vi "Update_Analized_CoorOverlay.vi"(4 "Index":i32, 5 "DLL/Vision":bool, 6 "Listbox In":string[][](array[string]), 7 "ROI Entry":T10={"vROIName"="", "vROIContour"={"Contour Type"=0, "ROI Type"=0, "Points"=[]}, "ProcessSetting"=[], "Analysis_Setting"={"PreProcess"=enum."*Algorithm*", "Parameter"=""}}, 8 "error in (no error)":errorcluster, 9 "Available Points In":refnum<vi>, 10 "AnalysisResult":variant, 11 "Image Refnum":refnum<vi>) -> (0 "error out":errorcluster, 3 "Listbox Out":string[][](array[string]))   [LabVIEW 2019]
uses:
  Control/CoordinateAnalysisSetting.ctl
  DLL/[Global] Image.vi
  Analysis/Controls/Parttern Match/Analysis_PatternMatch_ResultWithnumber.ctl
  Process/Controls/Process_Setting.ctl
  Analysis/Controls/Analysis_Setting.ctl
  Controls/Vision_DataEntry.ctl
  <vilib>/vision/Measure.llb/Edge New.ctl
  <vilib>/vision/Image Controls.llb/IMAQ Image.ctl
  Ctrl/VisionProcessName.ctl
panel:
  out "DLL Vision_Image":T1
  in  "Particle output cluster":T2
  in  "Clamp MAX output cluster":T3
  in  "Clamp output cluster":T5 {"?"."Rectangle"."Rotation" format="%.2f"; "?"."Rectangle"."Left" scale=0.0..1024.0; "?"."Rectangle"."Right" scale=0.0..1024.0}
  in  "Barcode 1D output cluster":T6
  in  "Edge Detectionoutput cluster":T8 {"?"."Edge Information"."Distance (Real-World)" format="%.2f"; "?"."Edge Information"."Location (Real-World)"."Y" format="%.2g"; "?"."Edge Information"."Location (Real-World)"."X" format="%.2f"; "?"."Edge Information"."Noise" format="%.2f"; "?"."Edge Information"."Location (Pixel)"."Y" format="%.2g"; "?"."Edge Information"."Location (Pixel)"."X" format="%.2f"; "?"."Edge Information"."Strength" format="%.2f"; "?"."Edge Information"."Distance (Pixel)" format="%.2f"}
  in  "Barcode 2D output cluster":T9
  in  "Vision_Image":T1(plugin-control)
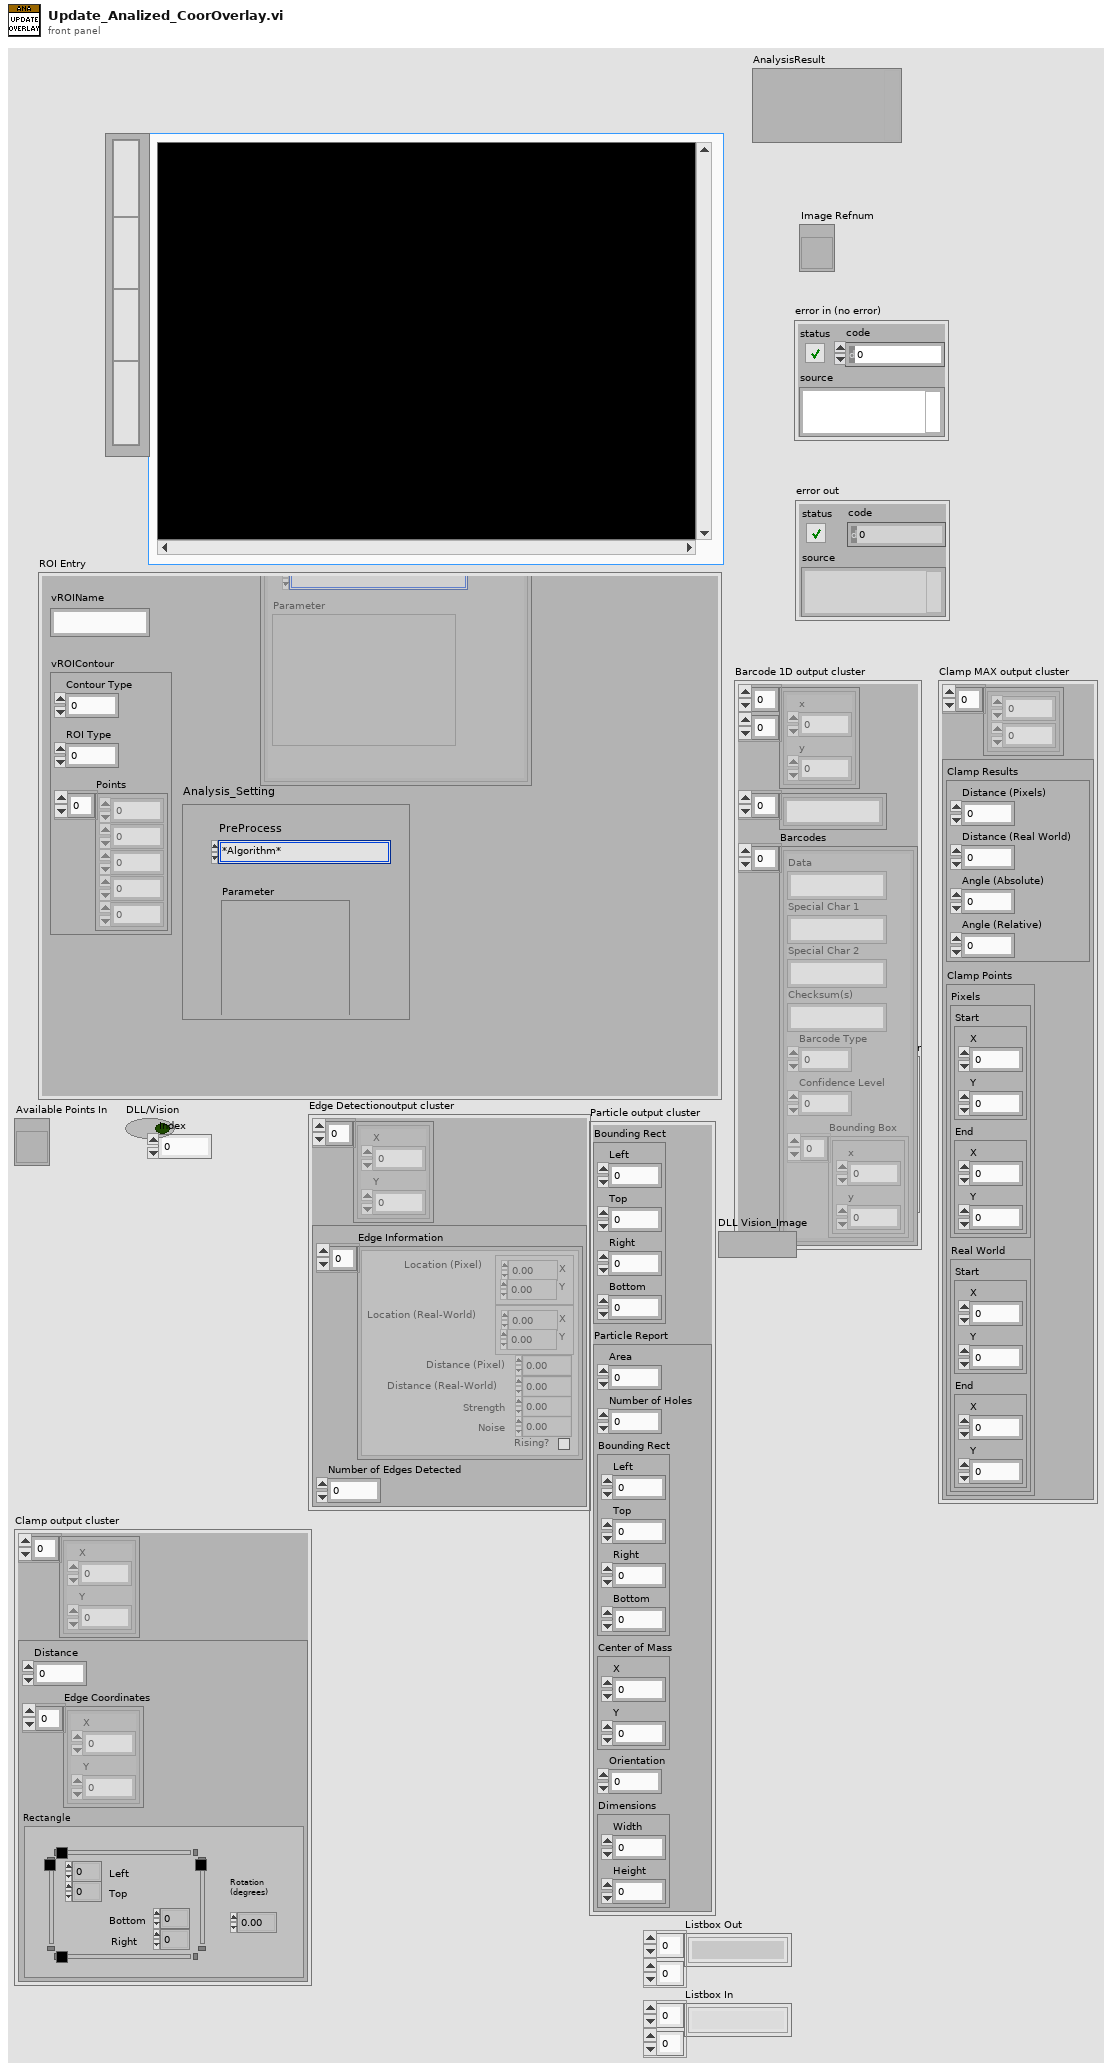
[diagram p1: front panel]
types:
  T1 = typedef "IMAQ Image.ctl" = refnum<image>
  T2 = cluster{"Bounding Rect":cluster{"Left":dbl, "Top":dbl, "Right":dbl, "Bottom":dbl}, "Particle Report":cluster{"Area":dbl, "Number of Holes":dbl, "Bounding Rect":cluster{"Left":dbl, "Top":dbl, "Right":dbl, "Bottom":dbl}, "Center of Mass":cluster{"X":dbl, "Y":dbl}, "Orientation":dbl, "Dimensions":cluster{"Width":dbl, "Height":dbl}}}
  T3 = cluster{cluster{dbl, dbl}[], cluster{"Clamp Results":cluster{"Distance (Pixels)":dbl, "Distance (Real World)":dbl, "Angle (Absolute)":dbl, "Angle (Relative)":dbl}, "Clamp Points":cluster{"Pixels ":cluster{"Start":cluster{"X":dbl, "Y":dbl}, "End":cluster{"X":dbl, "Y":dbl}}, "Real World":cluster{"Start":cluster{"X":dbl, "Y":dbl}, "End":cluster{"X":dbl, "Y":dbl}}}}}
  T4 = typedef "IMAQ Rectangle" = cluster{"Left":i32, "Top":i32, "Right":i32, "Bottom":i32, "Rotation":dbl}
  T5 = cluster{cluster{"X":sgl, "Y":sgl}[], cluster{"Distance":sgl, "Edge Coordinates":cluster{"X":sgl, "Y":sgl}[], "Rectangle":T4}}
  T6 = cluster{cluster{"x":sgl, "y":sgl}[][], string[], "Barcodes":cluster{"Data":string, "Special Char 1":string, "Special Char 2":string, "Checksum(s)":string, "Barcode Type":u32, "Confidence Level":sgl, "Bounding Box":cluster{"x":sgl, "y":sgl}[]}[]}
  T7 = typedef "Edge New.ctl" = cluster{"Location (Pixel)":cluster{"X":sgl, "Y":sgl}, "Location (Real-World)":cluster{"X":sgl, "Y":sgl}, "Distance (Pixel)":dbl, "Distance (Real-World)":dbl, "Strength":dbl, "Noise":dbl, "Rising?":bool}
  T8 = cluster{cluster{"X":sgl, "Y":sgl}[], cluster{"Edge Information":T7[], "Number of Edges Detected":i32}}
  T9 = cluster{"Data":string, cluster{"x":sgl, "y":sgl}[]}
  T10 = typedef "Vision_DataEntry.ctl" = cluster{"vROIName":string, "vROIContour":cluster{"Contour Type":u32, "ROI Type":u32, "Points":i32[]}, "ProcessSetting":T11[], "Analysis_Setting":T13}
  T11 = typedef "Process_Setting.ctl" = cluster{"Enum_PreProcess":T12, "Parameter":string}
  T12 = typedef "VisionProcessName.ctl" = enum16{"*CamParameter*", "CamAttributes", "*Preprocess*", "CG_Brightness", "C_Plane Extraction", "C_Threshold", "G_Lookup Table", "G_Threshold"}
  T13 = typedef "Analysis_Setting.ctl" = cluster{"PreProcess":T14, "Parameter":string}
  T14 = typedef "VisionProcessName.ctl" = enum16{"*CamParameter*", "CamAttributes", "*Preprocess*", "CG_Brightness", "C_Plane Extraction", "C_Threshold", "G_Lookup Table", "G_Threshold", "B_Image Inversion", "*Algorithm*", "CG_Histogram", "C_Color Matching", "C_Color Pattern Matching", "G_PatternMatch", "CG_Find Straight Edge", "CG_Adv. Find Straight Edge", "CG_Find Circular Edge", "G_Max Clamp", "G_Clamp (Rake)", "G_Pattern Matching"}
  T15 = typedef "CoordinateAnalysisSetting.ctl" = cluster{"Analysis_Type":enum16{"PatternMatch", "Straight Edge"}, "ROI ":T16, "Parameter":variant, "Step Result":variant, "AnalysisStepName":string, "CoordinateUse":bool}
  T16 = typedef "ROI Descriptor" = cluster{"Global Rectangle":i32[], "Contours":cluster{"ID":enum32{"External", "Internal"}, "Type":u32, "Coordinates":i32[]}[]}
  T17 = typedef "Analysis_Type.ctl" = u16
  T18 = typedef "Analysis_PatternMatch_ResultWithnumber.ctl" = cluster{"numbers":i32, "results":cluster{"ROI Descriptor out":T16, "Point":T19, "Angle":sgl, "Score":sgl, "Real World Coordinates":cluster{"X":sgl, "Y":sgl}, "Rectangle":T4}[]}
  T19 = typedef "IMAQ Point" = cluster{"X":sgl, "Y":sgl}
  T20 = cluster{"Point1 (Pixels)":cluster{"X":sgl, "Y":sgl}, "Point2 (Pixels)":cluster{"X":sgl, "Y":sgl}, "Point1 (Real-World)":cluster{"X":sgl, "Y":sgl}, "Point2 (Real-World)":cluster{"X":sgl, "Y":sgl}, "Angle (Pixel)":dbl, "Angle (Real-World)":dbl, "Score":dbl, "Straightness":dbl, "Average SNR (db)":dbl, "Calibration Valid":bool}[]
  T21 = cluster{"ROI Descriptor out":T16, "Point":T19, "Angle":sgl, "Score":sgl, "Real World Coordinates":cluster{"X":sgl, "Y":sgl}, "Rectangle":T4}[]
  T22 = cluster{"Left":dbl, "Top":dbl, "Right":dbl, "Bottom":dbl}
  T23 = cluster{"ROI Descriptor out":cluster{"Global Rectangle":i32[], "Contours":cluster{"ID":enum32{"External", "Internal"}, "Type":u32, "Coordinates":i32[]}[]}, "Output value":dbl}
  T24 = cluster{"Global Rectangle":i32[], "Contours":cluster{"ID":enum32{"External", "Internal"}, "Type":u32, "Coordinates":i32[]}[]}
  T25 = cluster{"ID":enum32{"External", "Internal"}, "Type":u32, "Coordinates":i32[]}[]
  T26 = cluster{"ID":enum32{"External", "Internal"}, "Type":u32, "Coordinates":i32[]}
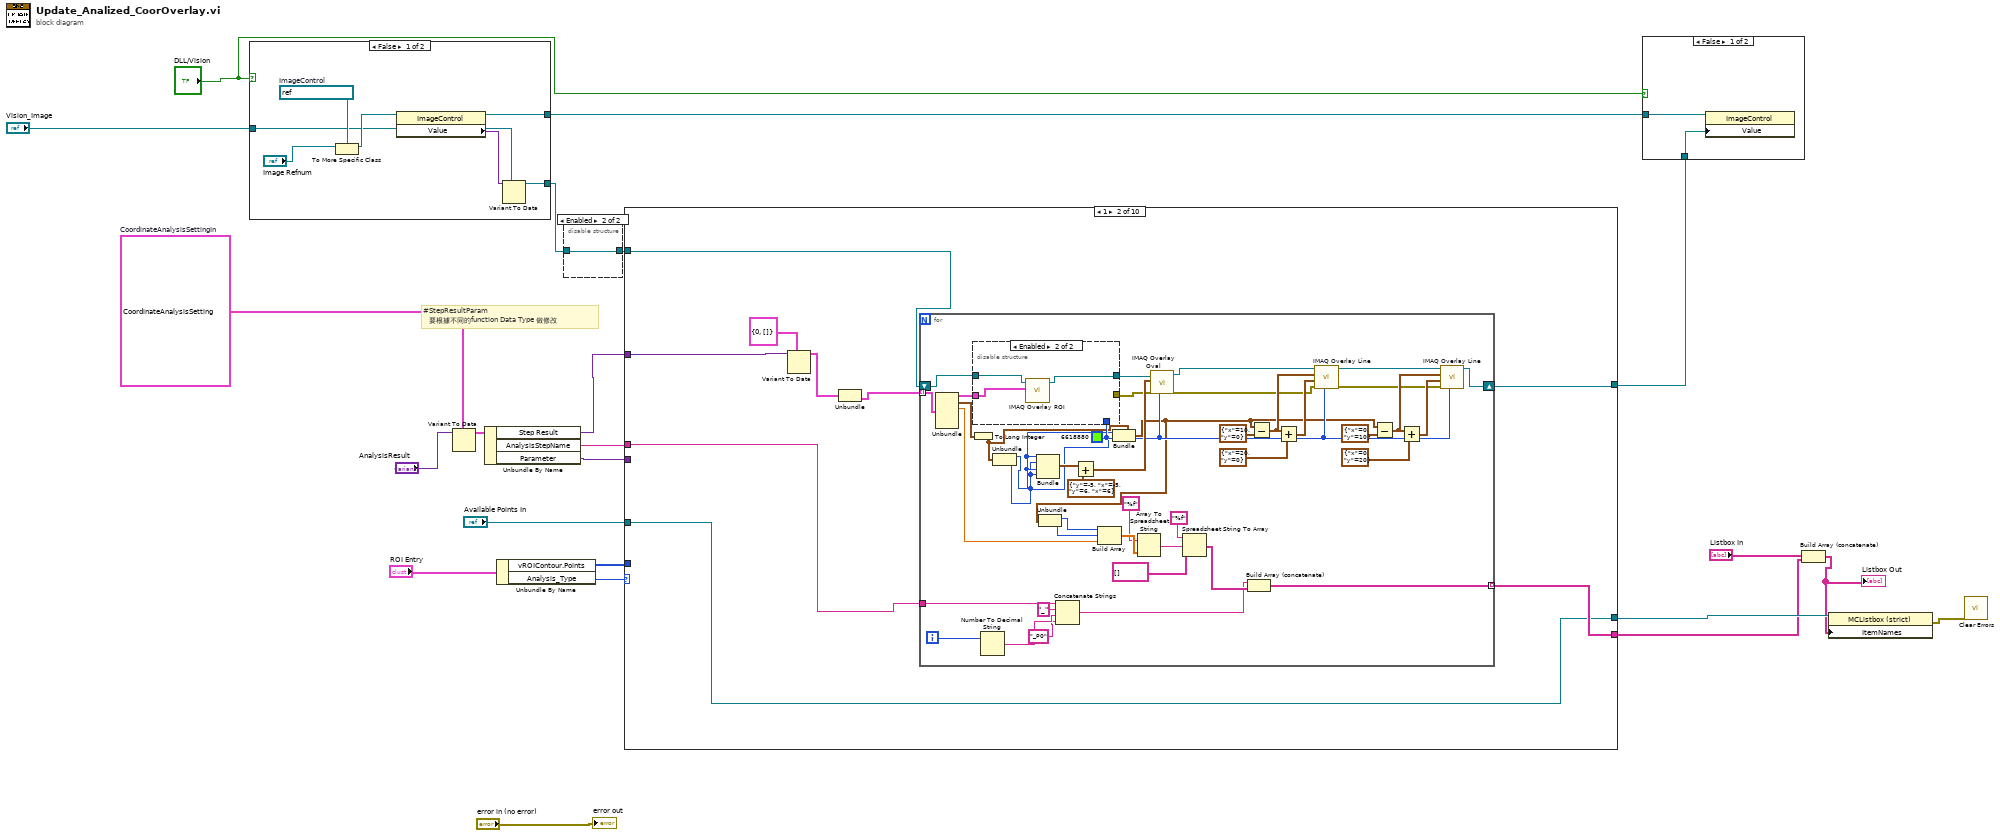
[diagram p0: block diagram]
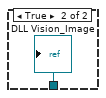
[diagram p2: hidden frame]
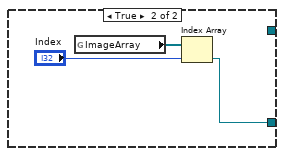
[diagram p3: hidden frame]
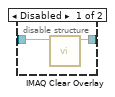
[diagram p4: hidden frame]
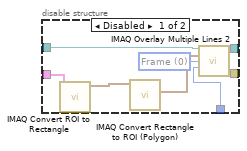
[diagram p6: hidden frame]
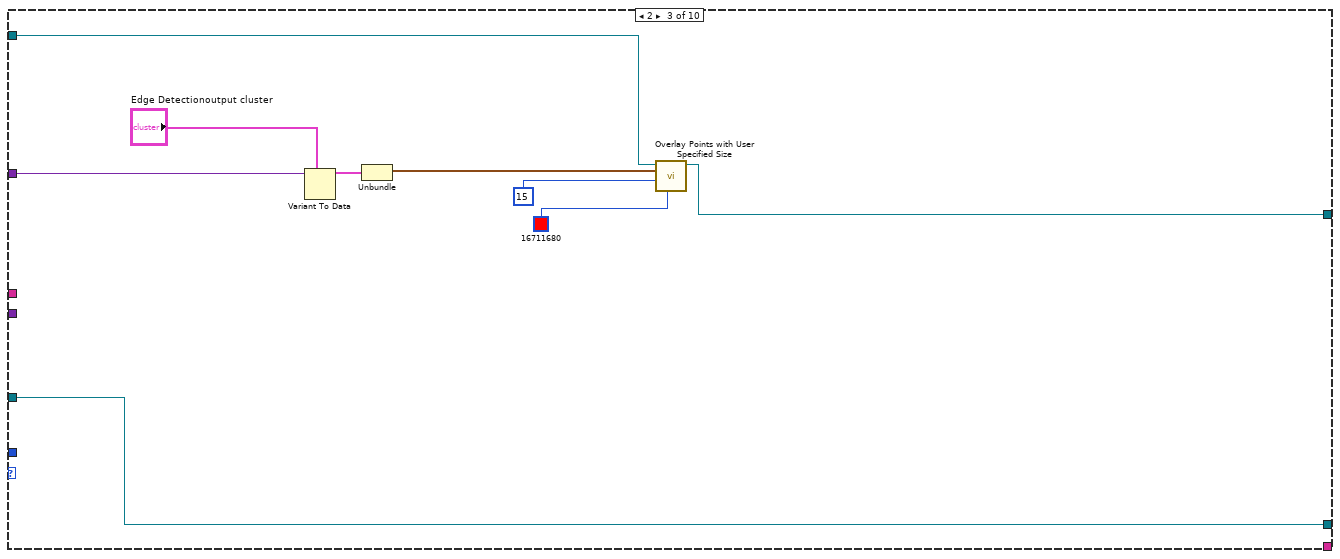
[diagram p7: hidden frame]
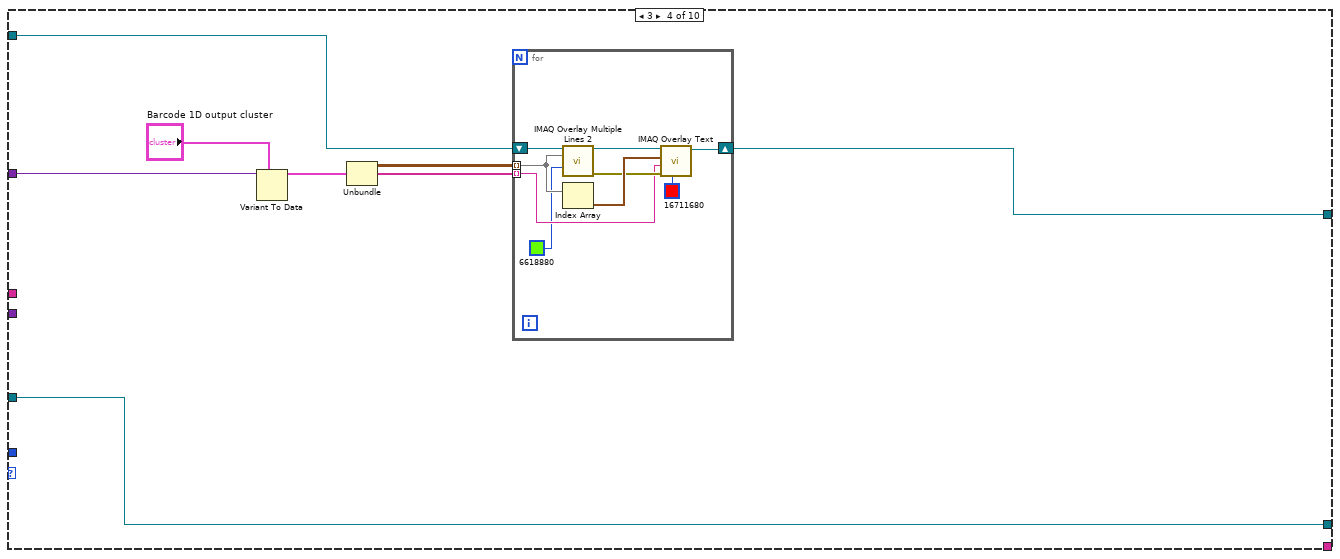
[diagram p8: hidden frame]
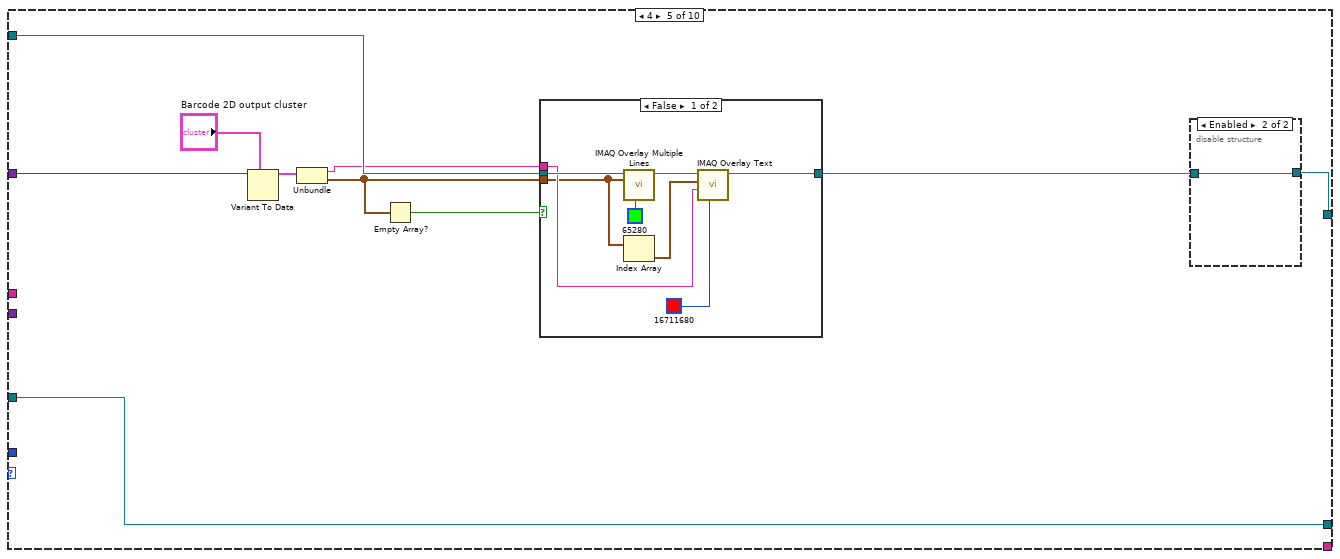
[diagram p9: hidden frame]
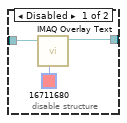
[diagram p11: hidden frame]
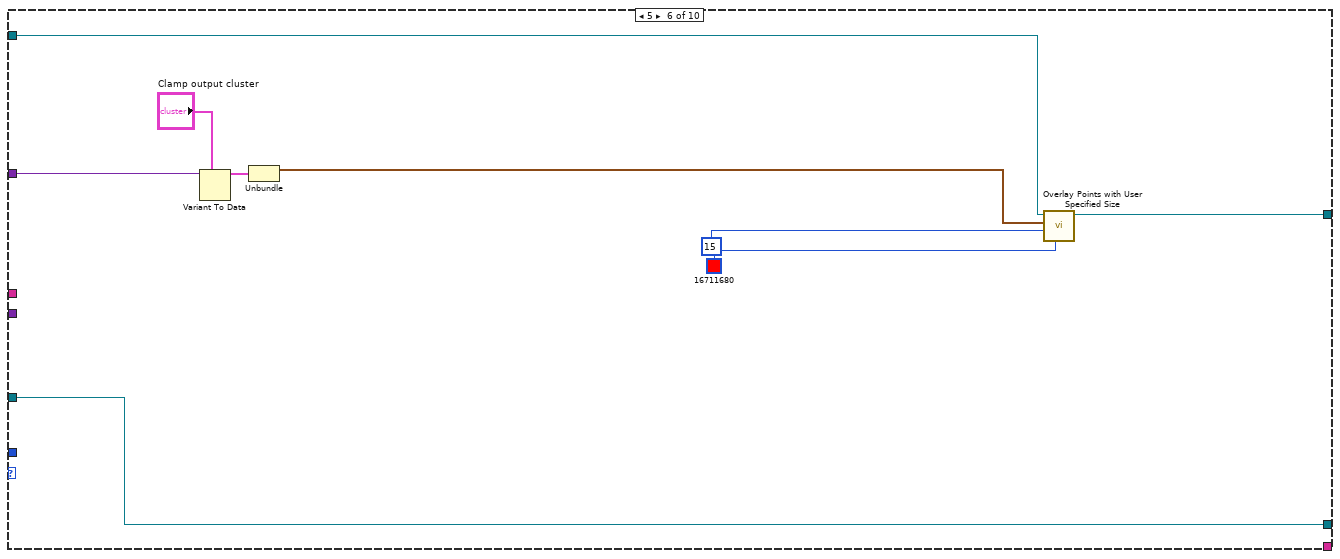
[diagram p12: hidden frame]
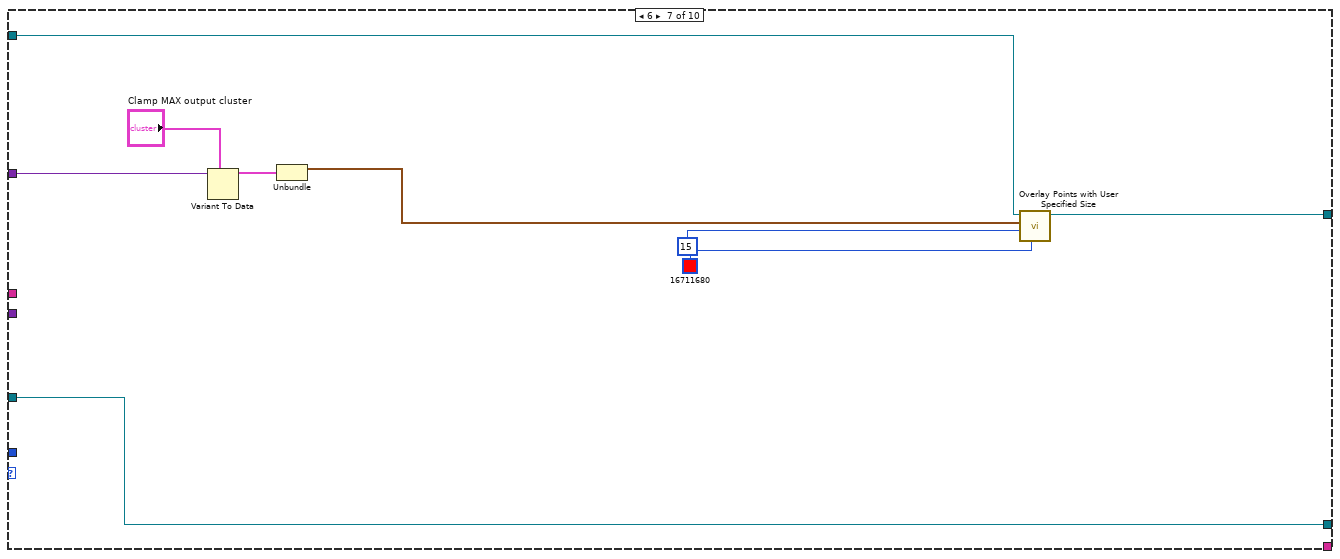
[diagram p13: hidden frame]
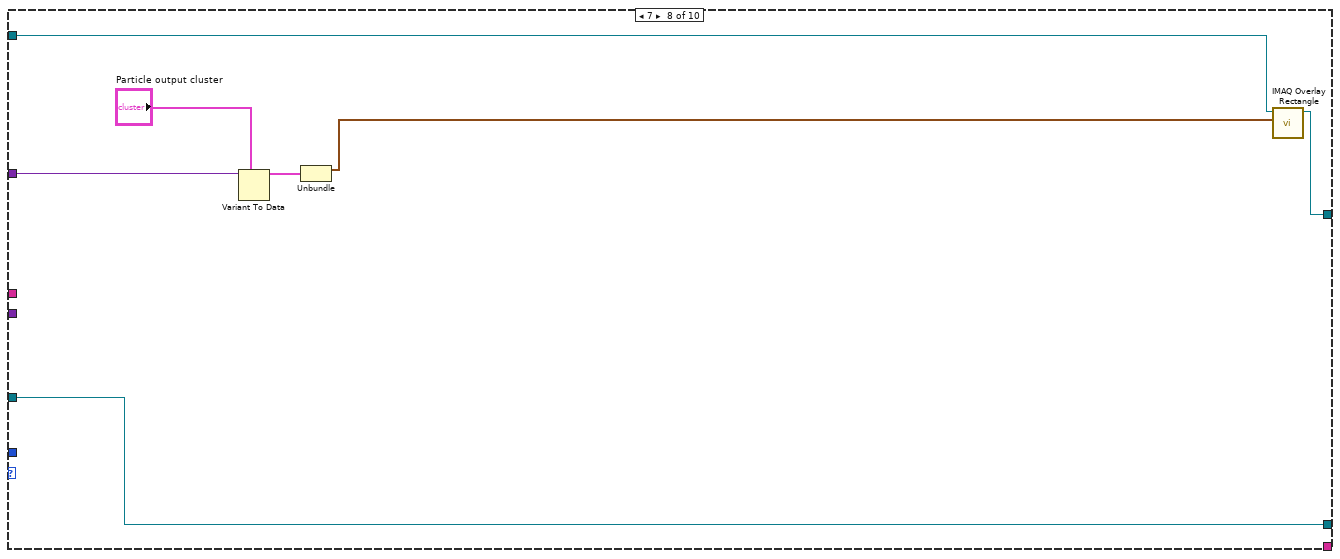
[diagram p14: hidden frame]
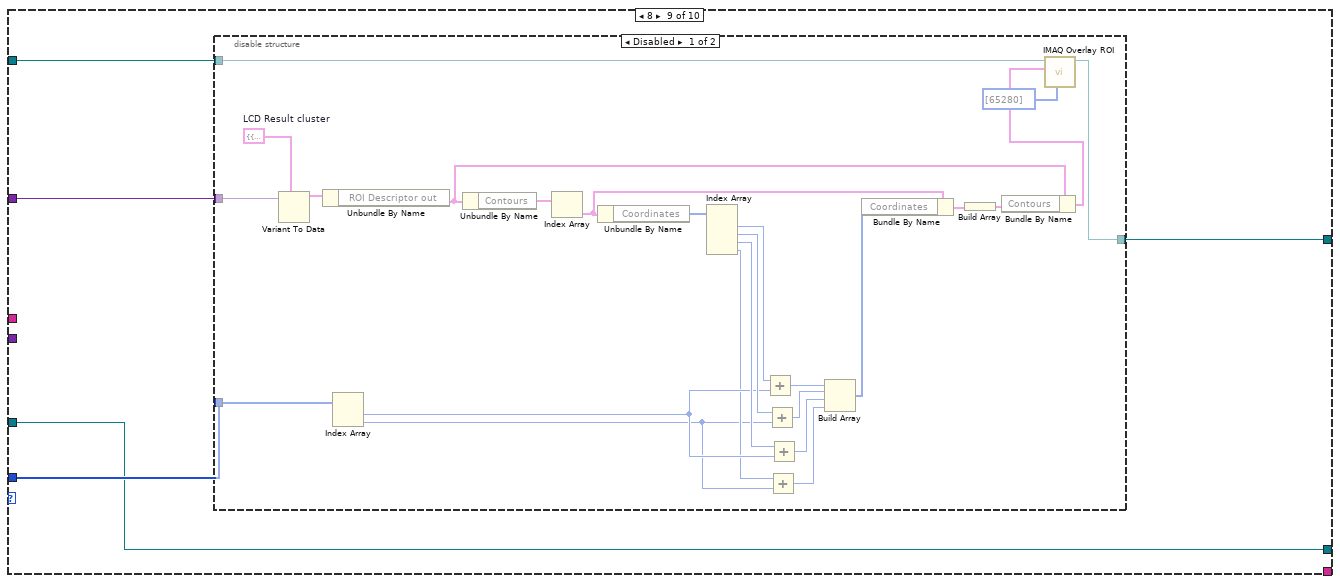
[diagram p15: hidden frame]
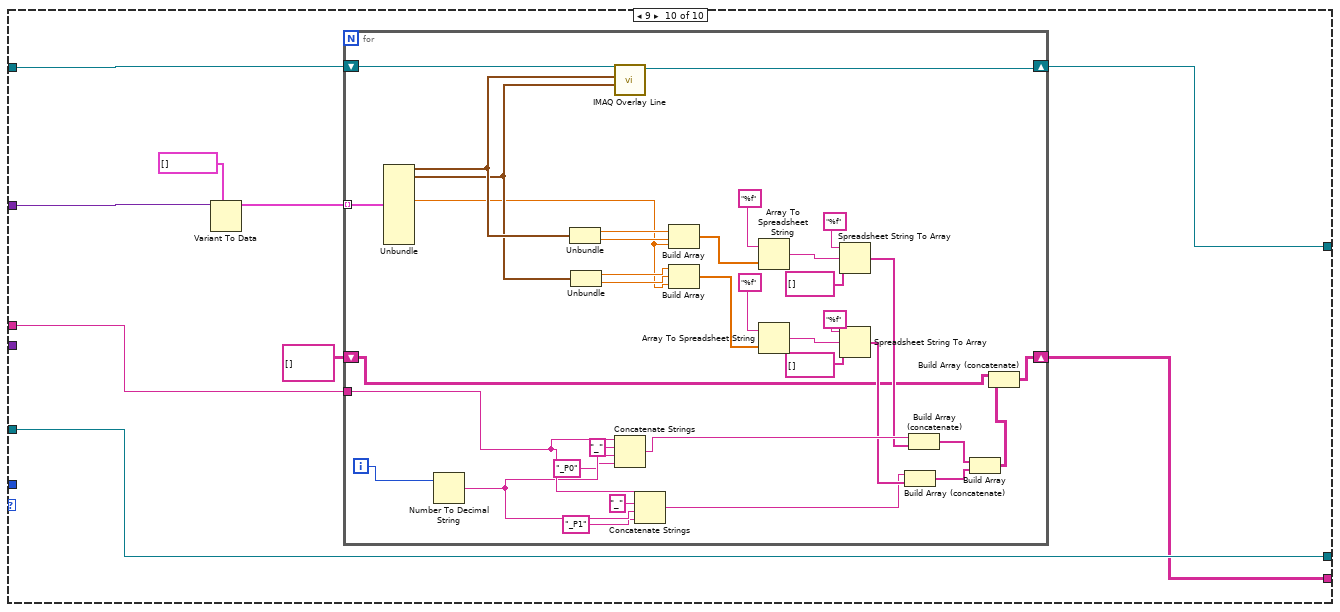
[diagram p17: hidden frame]
diagram:
  w12 = T15 {"Analysis_Type"=enum."PatternMatch", "ROI "={"Global Rectangle"=[], "Contours"=[]}, "Parameter"=variant, "Step Result"=variant, "AnalysisStepName"="", "CoordinateUse"=FALSE}  # CoordinateAnalysisSettingIn
  # "#StepResultParam\n   要根據不同的function Data Type 做修改"
  n1 = case shown="False" "DLL/Vision" {
    tunnel: [w26 _] -> w22
    tunnel: "Vision_Image" -> [w25 _]
    tunnel: [w23 w30] -> w20
    frame False {
      w28 = refnum<vi> refnum  # ImageControl
      n2 = To More Specific Class(target class=w28, reference="Image Refnum") -> (specific class reference=w27:refnum<vi>)  [unwired: 1 in, 1 out]
      n3 = property class="ImageControl"(reference=w27) -> (reference out=w26:refnum<vi>, "Value"=w24:variant)  [unwired: 1 in, 1 out]
      n4 = Variant To Data(type=w25, Variant=w24) -> (data=w23:T1)  [unwired: 1 in, 1 out]
    }
    frame True {
      n5 = global read "[Global] Image.vi" "ImageArray"() -> (w32:T1[])
      n6 = Index Array(array=w32, index="Index") -> (element=w30:T1)
    }
  }
  n7 = Variant To Data(type=w12, Variant="AnalysisResult") -> (data=w11:T15)  [unwired: 1 in, 1 out]
  n8 = Unbundle By Name(w11) -> ("Step Result"=w10:variant, "AnalysisStepName"=w9:string, "Parameter"=w4:variant)
  n9 = Unbundle By Name("ROI Entry") -> ("vROIContour.Points"=w16:i32[], "Analysis_Type"=w15:T17)
  n10 = disable-structure shown="Enabled" {
    disable-tunnel: w20 -> [w34 w35]
    disable-tunnel: [w33 w35] -> w19
    frame Disabled {
      n11 = call "IMAQ Clear Overlay"("Image"=w34) -> ("Image Out"=w33:T1)  [unwired: 9 in, 1 out]
    }
    frame Enabled {
    }
  }
  n12 = case shown="1" w15 {
    tunnel: w10 -> [_ w46 w109 w117 w136 w158 w167 w174 w179 w209]
    tunnel: w16 -> [_ _ _ _ _ _ _ _ w176 _]
    tunnel: w19 -> [w37 w45 w108 w113 w133 w155 w164 w173 w178 w210]
    tunnel: [w37 w44 w106 w111 w131 w154 w163 w172 w177 w206] -> w18
    tunnel: "Available Points In" -> [w36 w40 w101 w110 w127 w150 w159 w168 w175 w213]
    tunnel: w9 -> [_ w42 _ _ _ _ _ _ _ w208]
    tunnel: [_ w41 _ _ _ _ _ _ _ w207] -> w7
    tunnel: [w36 w40 w101 w110 w127 w150 w159 w168 w175 w213] -> w8
    tunnel: w4 -> [_ _ _ _ _ _ _ _ _ _]
    frame 0, Default {
    }
    frame 1 {
      n13 = Variant To Data(type=T18 {"numbers"=0, "results"=[]} ("PatternMatchResult"), Variant=w46) -> (data=w43:T18)  [unwired: 1 in, 1 out]
      n14 = Unbundle(w43) -> ("results"=w38:T21)  [unwired: 1 out]
      n15 = for {
        tunnel: w38 -> [w88] mode=indexing
        tunnel: w42 -> [w57]
        tunnel: [w58] -> w41 mode=indexing
        shift-right: [w69] -> w44
        shift-left: w45 -> [w89]
        i -> [w56]
        w54 = u32 6618880 ("Color")
        n16 = Unbundle(w88) -> ("ROI Descriptor out"=w87:T16, "Point"=w68:T19, "Angle"=w65:sgl)  [unwired: 3 out]
        n17 = To Long Integer(number=w68) -> (32bit integer=w53:cluster{"X":i32, "Y":i32})
        n18 = disable-structure shown="Enabled" {
          disable-tunnel: w89 -> [w97 w100]
          disable-tunnel: w87 -> [w93 w99]
          disable-tunnel: [w92 w98] -> w86
          disable-tunnel: [w91 _] -> w72
          disable-tunnel: w54 -> [w90 _]
          frame Disabled {
            w94 = u32 0 items=["Frame", "Fill"] ("Drawing Mode (Frame)")
            n19 = call "IMAQ Convert ROI to Rectangle"("ROI Descriptor"=w93) -> ("Rectangle"=w95:T4)  [unwired: 8 in, 1 out]
            n20 = call "IMAQ Convert Rectangle to ROI (Polygon)"("Rectangle"=w95) -> ("Rectangle Points"=w96:T19[])  [unwired: 7 in, 2 out]
            n21 = call "IMAQ Overlay Multiple Lines 2"("Image"=w97, "Line End Points"=w96, "Drawing Mode (Frame)"=w94, "Color"=w90) -> ("Image Out"=w92:T1, "error out"=w91:errorcluster)  [unwired: 10 in]
          }
          frame Enabled {
            n22 = call "IMAQ Overlay ROI"("ROI Descriptor"=w99, "Image"=w100) -> ("Image Out"=w98:T1)  [unwired: 8 in, 1 out]
          }
        }
        n23 = Number To Decimal String(number=w56) -> (decimal integer string=w50:string)  [unwired: 1 in]
        n24 = Unbundle(w53) -> ("X"=w48:i32, "Y"=w47:i32)
        n25 = Bundle("X"=w48, "Y"=w47, "X"=w48, "Y"=w47) -> (w85:cluster{"X":i32, "Y":i32, "X":i32, "Y":i32})  [unwired: 1 out]
        n26 = Concatenate Strings(w57, "_" ("string"), w50, "_P0" ("string")) -> (w55:string)
        n27 = Add(x=w85, y=cluster{"y":i32, "x":i32, "y":i32, "x":i32} {"y"=-5, "x"=-5, "y"=6, "x"=6}) -> (x+y=w83:cluster{i32, i32, i32, i32})
        n28 = Bundle(cluster=w53, "X"=w48, "Y"=w47) -> (w52:cluster{"X":i32, "Y":i32})
        n29 = Unbundle(w52) -> ("X"=w67:i32, "Y"=w66:i32)
        n30 = Build Array(w67, w66, w65) -> (w64:sgl[])
        n31 = Array To Spreadsheet String(array=w64, 3:"%f" ("format string")) -> (spreadsheet string=w62:string)  [unwired: 1 in]
        n32 = call "IMAQ Overlay Oval"("Color"=w54, "error in (no error)"=w72, "Bounding Rectangle"=w83, "Image"=w86) -> ("error out"=w71:errorcluster, "Image Out"=w70:T1)  [unwired: 6 in]
        n33 = Spreadsheet String To Array(format string="%f", spreadsheet string=w62, array type (2D Dbl)=string[] []) -> (array=w59:string[])  [unwired: 1 in]
        n34 = Build Array (concatenate)(w55, w59) -> (w58:string[])
        n35 = Subtract(x=w52, y=cluster{"x":i32, "y":i32} {"x"=10, "y"=0}) -> (x-y=w81:cluster{i32, i32})
        n36 = Add(x=w81, y=cluster{"x":i32, "y":i32} {"x"=20, "y"=0}) -> (x+y=w79:cluster{i32, i32})
        n37 = call "IMAQ Overlay Line"("Color"=w54, "error in (no error)"=w71, "End Point"=w79, "Start Point"=w81, "Image"=w70) -> ("error out"=w73:errorcluster, "Image Out"=w74:T1)  [unwired: 1 in, 4 out]
        n38 = Subtract(x=w52, y=cluster{"x":i32, "y":i32} {"x"=0, "y"=10}) -> (x-y=w77:cluster{i32, i32})
        n39 = Add(x=w77, y=cluster{"x":i32, "y":i32} {"x"=0, "y"=20}) -> (x+y=w78:cluster{i32, i32})
        n40 = call "IMAQ Overlay Line"("Color"=w54, "error in (no error)"=w73, "End Point"=w78, "Start Point"=w77, "Image"=w74) -> ("Image Out"=w69:T1)  [unwired: 1 in, 5 out]
      }
    }
    frame 2 {
      n41 = Variant To Data(type="Edge Detectionoutput cluster", Variant=w109) -> (data=w103:T8)  [unwired: 1 in, 1 out]
      n42 = Unbundle(w103) -> (w102:cluster{"X":sgl, "Y":sgl}[])  [unwired: 1 out]
      n43 = call "Overlay Points with User Specified Size.vi"("Color"=u32 16711680, "Point Diameter (5)"=u32 15, "Points"=w102, "Image In"=w108) -> ("Image Out"=w106:T1)  [unwired: 6 in, 1 out]
    }
    frame 3 {
      n44 = Variant To Data(type="Barcode 1D output cluster", Variant=w117) -> (data=w115:T6)  [unwired: 1 in, 1 out]
      n45 = Unbundle(w115) -> (w114:cluster{"x":sgl, "y":sgl}[][], w112:string[])  [unwired: 1 out]
      n46 = for {
        tunnel: w114 -> [w121] mode=indexing
        shift-right: [w119] -> w111
        shift-left: w113 -> [w122]
        tunnel: w112 -> [w120] mode=indexing
        n47 = call "IMAQ Overlay Multiple Lines 2"("Image"=w122, "Line End Points"=w121, "Color"=u32 6618880) -> ("Image Out"=w123:T1, "error out"=w125:errorcluster)  [unwired: 11 in]
        n48 = Index Array(array=w121) -> (element=w126:cluster{"x":sgl, "y":sgl})  [unwired: 1 in]
        n49 = call "IMAQ Overlay Text"("Text Color (black)"=u32 16711680, "error in (no error)"=w125, "String"=w120, "Origin"=w126, "Image"=w123) -> ("Image Out"=w119:T1)  [unwired: 5 in, 1 out]
      }
    }
    frame 4 {
      n50 = Variant To Data(type="Barcode 2D output cluster", Variant=w136) -> (data=w134:T9)  [unwired: 1 in, 1 out]
      n51 = Unbundle(w134) -> ("Data"=w128:string, w130:cluster{"x":sgl, "y":sgl}[])
      n52 = Empty Array?(array=w130) -> (empty?=w129:bool)
      n53 = case shown="False" w129 {
        tunnel: w133 -> [w143 w145]
        tunnel: [w141 w145] -> w132
        tunnel: w130 -> [w139 _]
        tunnel: w128 -> [w140 _]
        frame False {
          n54 = call "IMAQ Overlay Multiple Lines"("Color"=u32 65280, "Line End Points"=w139, "Image"=w143) -> ("Image Out"=w142:T1)  [unwired: 7 in, 1 out]
          n55 = Index Array(array=w139) -> (element=w138:cluster{"x":sgl, "y":sgl})  [unwired: 1 in]
          n56 = call "IMAQ Overlay Text"("Text Color (black)"=u32 16711680, "String"=w140, "Origin"=w138, "Image"=w142) -> ("Image Out"=w141:T1)  [unwired: 6 in, 1 out]
        }
        frame True {
        }
      }
      n57 = disable-structure shown="Enabled" {
        disable-tunnel: w132 -> [w147 w149]
        disable-tunnel: [w146 w149] -> w131
        frame Disabled {
          n58 = call "IMAQ Overlay Text"("Text Color (black)"=u32 16711680, "Image"=w147) -> ("Image Out"=w146:T1)  [unwired: 8 in, 1 out]
        }
        frame Enabled {
        }
      }
    }
    frame 5 {
      n59 = Variant To Data(type="Clamp output cluster", Variant=w158) -> (data=w152:T5)  [unwired: 1 in, 1 out]
      n60 = Unbundle(w152) -> (w151:cluster{"X":sgl, "Y":sgl}[])  [unwired: 1 out]
      n61 = call "Overlay Points with User Specified Size.vi"("Color"=u32 16711680, "Point Diameter (5)"=u32 15, "Points"=w151, "Image In"=w155) -> ("Image Out"=w154:T1)  [unwired: 6 in, 1 out]
    }
    frame 6 {
      n62 = Variant To Data(type="Clamp MAX output cluster", Variant=w167) -> (data=w161:T3)  [unwired: 1 in, 1 out]
      n63 = Unbundle(w161) -> (w160:cluster{dbl, dbl}[])  [unwired: 1 out]
      n64 = call "Overlay Points with User Specified Size.vi"("Color"=u32 16711680, "Point Diameter (5)"=u32 15, "Points"=w160, "Image In"=w164) -> ("Image Out"=w163:T1)  [unwired: 6 in, 1 out]
    }
    frame 7 {
      n65 = Variant To Data(type="Particle output cluster", Variant=w174) -> (data=w170:T2)  [unwired: 1 in, 1 out]
      n66 = Unbundle(w170) -> ("Bounding Rect"=w169:T22)  [unwired: 1 out]
      n67 = call "IMAQ Overlay Rectangle"("Rectangle"=w169, "Image"=w173) -> ("Image Out"=w172:T1)  [unwired: 8 in, 1 out]
    }
    frame 8 {
      n68 = disable-structure shown="Disabled" {
        disable-tunnel: w179 -> [w204 _]
        disable-tunnel: w178 -> [w202 _]
        disable-tunnel: [w200 _] -> w177
        disable-tunnel: w176 -> [w199 _]
        frame Disabled {
          w203 = T23 {"ROI Descriptor out"={"Global Rectangle"=[], "Contours"=[]}, "Output value"=0.0}  # LCD Result cluster
          n69 = Variant To Data(type=w203, Variant=w204) -> (data=w182:T23)  [unwired: 1 in, 1 out]
          n70 = Unbundle By Name(w182) -> ("ROI Descriptor out"=w181:T24)
          n71 = Index Array(array=w199) -> (element #1=w193:i32, element #2=w191:i32)  [unwired: 2 in]
          n72 = Unbundle By Name(w181) -> ("Contours"=w198:T25)
          n73 = Index Array(array=w198) -> (element=w186:T26)  [unwired: 1 in]
          n74 = Unbundle By Name(w186) -> ("Coordinates"=w197:i32[])
          n75 = Index Array(array=w197) -> (element #1=w196:i32, element #2=w195:i32, element #3=w194:i32, element #4=w192:i32)  [unwired: 4 in]
          n76 = Add(x=w196, y=w193) -> (x+y=w190:i32)
          n77 = Add(x=w195, y=w191) -> (x+y=w189:i32)
          n78 = Add(x=w192, y=w191) -> (x+y=w187:i32)
          n79 = Add(x=w194, y=w193) -> (x+y=w188:i32)
          n80 = Build Array(w190, w189, w188, w187) -> (w185:i32[])
          n81 = Bundle By Name(cluster=w186, "Coordinates"=w185) -> (w184:T26)
          n82 = Build Array(w184) -> (w183:T25)
          n83 = Bundle By Name(cluster=w181, "Contours"=w183) -> (w180:T24)
          n84 = call "IMAQ Overlay ROI"("Colors (Green)"=u32[] [65280], "ROI Descriptor"=w180, "Image"=w202) -> ("Image Out"=w200:T1)  [unwired: 7 in, 1 out]
        }
        frame Enabled {
        }
      }
    }
    frame 9 {
      n85 = Variant To Data(type=T20 [] ("Straight Edge Cluster Array"), Variant=w209) -> (data=w212:T20)  [unwired: 1 in, 1 out]
      n86 = for {
        tunnel: w212 -> [w249] mode=indexing
        shift-right: [w247] -> w206
        shift-left: w210 -> [w248]
        tunnel: w208 -> [w225]
        shift-right: [w218] -> w207
        shift-left: string[][] [] -> [w220]
        i -> [w237]
        n87 = Unbundle(w249) -> ("Point1 (Pixels)"=w246:cluster{"X":sgl, "Y":sgl}, "Point2 (Pixels)"=w245:cluster{"X":sgl, "Y":sgl}, "Angle (Pixel)"=w232:dbl)  [unwired: 7 out]
        n88 = Number To Decimal String(number=w237) -> (decimal integer string=w224:string)  [unwired: 1 in]
        n89 = Unbundle(w246) -> ("X"=w244:sgl, "Y"=w243:sgl)
        n90 = Unbundle(w245) -> ("X"=w234:sgl, "Y"=w233:sgl)
        n91 = call "IMAQ Overlay Line"("End Point"=w245, "Start Point"=w246, "Image"=w248) -> ("Image Out"=w247:T1)  [unwired: 7 in, 1 out]
        n92 = Concatenate Strings(w225, "_" ("string"), w224, "_P0" ("string")) -> (w236:string)
        n93 = Concatenate Strings(w225, "_" ("string"), w224, "_P1" ("string")) -> (w223:string)
        n94 = Build Array(w244, w243, w232) -> (w238:dbl[])
        n95 = Build Array(w234, w233, w232) -> (w227:dbl[])
        n96 = Array To Spreadsheet String(array=w238, 3:"%f" ("format string")) -> (spreadsheet string=w241:string)  [unwired: 1 in]
        n97 = Array To Spreadsheet String(array=w227, 3:"%f" ("format string")) -> (spreadsheet string=w229:string)  [unwired: 1 in]
        n98 = Spreadsheet String To Array(format string="%f", spreadsheet string=w241, array type (2D Dbl)=string[] []) -> (array=w235:string[])  [unwired: 1 in]
        n99 = Spreadsheet String To Array(format string="%f", spreadsheet string=w229, array type (2D Dbl)=string[] []) -> (array=w226:string[])  [unwired: 1 in]
        n100 = Build Array (concatenate)(w223, w226) -> (w221:string[])
        n101 = Build Array (concatenate)(w236, w235) -> (w222:string[])
        n102 = Build Array(w222, w221) -> (w219:string[][])
        n103 = Build Array (concatenate)(w220, w219) -> (w218:string[][])
      }
    }
  }
  n104 = case shown="False" "DLL/Vision" {
    tunnel: w22 -> [w251 _]
    tunnel: w18 -> [w250 w252]
    frame False {
      n105 = property class="ImageControl"(reference=w251, "Value"=w250) -> ()  [unwired: 1 in, 2 out]
    }
    frame True {
      "DLL Vision_Image" <- w252
    }
  }
  n106 = Build Array (concatenate)("Listbox In", w7) -> (w6:string[][])
  "Listbox Out" <- w6
  n107 = property class="MCListbox (strict)"(reference=w8, "ItemNames"=w6) -> (error out=w2:errorcluster)  [unwired: 1 in, 1 out]
  n108 = call <vilib>:"Clear Errors.vi"("error in (no error)"=w2) -> ()  [unwired: 5 in, 2 out]
  "error out" <- "error in (no error)"
